vi "Get Impulse.vi"(8 "error in (no error)":errorcluster, 10 "index":i32, 11 "Impulse Manager in":refnum<class "Impulse Manager.lvclass">) -> (0 "error out":errorcluster, 2 "Reference out":T1, 3 "Impulse Manager out":refnum<class "Impulse Manager.lvclass">)   [LabVIEW 2013, in "Impulse Manager.lvclass"]
uses:
  Impulse Manager.lvclass
  Impulse Data/Instance handle.ctl
  Impulse Data/Impulse Data.lvclass
  Impulse Manager.lvclass/Impulse Manager.ctl
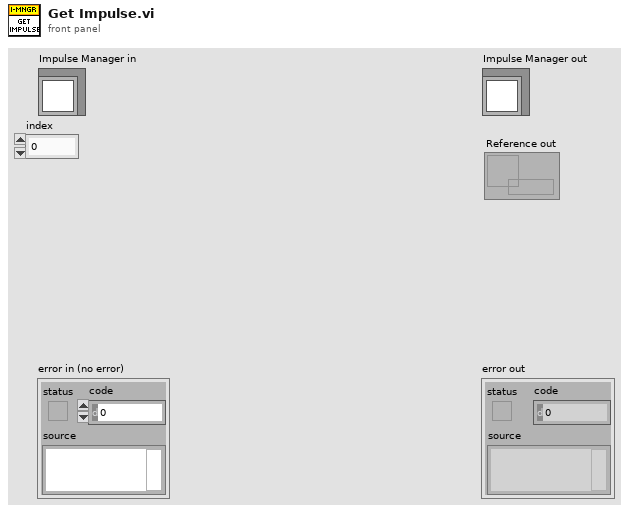
[diagram p1: front panel]
types:
  T1 = typedef "Impulse Data.lvclass/Instance handle.ctl" = refnum<data-value>
  T2 = typedef "core.lvlib/TD_Impulse Parameter.ctl" = cluster{"Color":u32, "Visible":bool, "Channel":u16, "Invert":bool, "Desaccade":bool, "Offset":dbl, "Gain":dbl}[]
  T3 = cluster{"Color":u32, "Visible":bool, "Channel":u16, "Invert":bool, "Desaccade":bool, "Offset":dbl, "Gain":dbl}
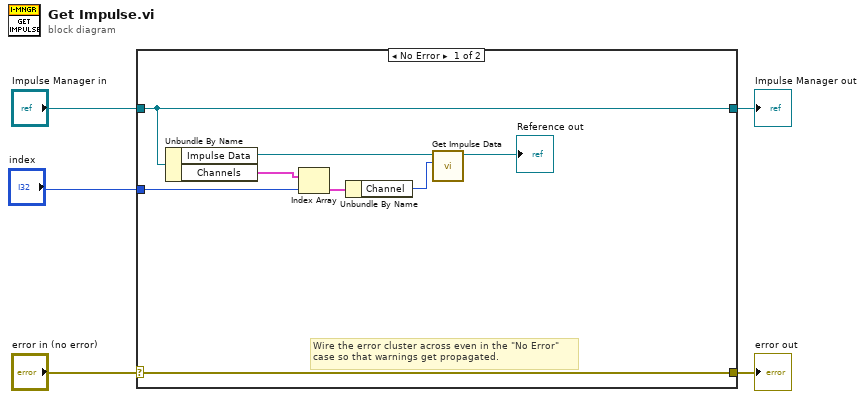
[diagram p0: block diagram]
diagram:
  n1 = case shown="No Error" "error in (no error)" {
    selector: "error in (no error)" -> [w13 w15]
    tunnel: [w13 w15] -> w4
    tunnel: [w7 w14] -> w2
    tunnel: "Impulse Manager in" -> [w7 w14]
    tunnel: "index" -> [w8 _]
    frame No Error {
      # "Wire the error cluster across even in the \"No Error\"\ncase so that warnings get propagated."
      n2 = Unbundle By Name(w7) -> ("Impulse Data"=w10:T1, "Channels"=w9:T2)
      n3 = Index Array(array=w9, index=w8) -> (element=w11:T3)
      n4 = Unbundle By Name(w11) -> ("Channel"=w12:u16)
      n5 = call "Get Impulse Data.vi"("Channel"=w12, "Reference in"=w10) -> ("Reference out"=→"Reference out":T1)  [unwired: 8 in, 1 out]
    }
    frame Error {
    }
  }
  "error out" <- w4
  "Impulse Manager out" <- w2
